vi "Find Ni-Scope digitizers.vi"(8 "Error In":errorcluster) -> (0 "Error Out":errorcluster, 2 "Device names out":string[](array[string]), 3 "Digitizers out":refnum<class "Pulse Driver.lvclass">[](array[class]))   [LabVIEW 2016, in "Ni-Scope Digitizer.lvclass"]
uses:
  Ni-Scope Digitizer.lvclass
  Instruments/Pulse Driver/Pulse Driver.lvclass
  C:/github/NHMFL_Core/Libraries/Instruments/Pulse Driver/Pulse Driver.lvclass
  Ni-Scope Digitizer.lvclass/Ni-Scope Digitizer.ctl
  Write Device name.vi
  <instrlib>/niModInst/niModInst Get Installed Device Attribute (String).vi
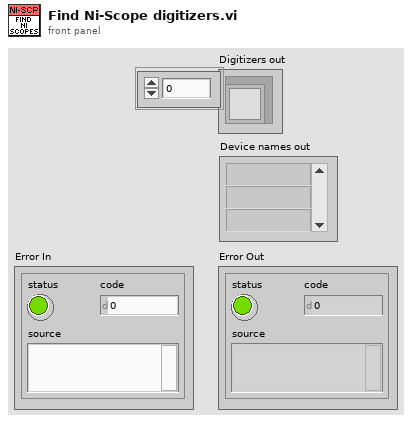
[diagram p1: front panel]
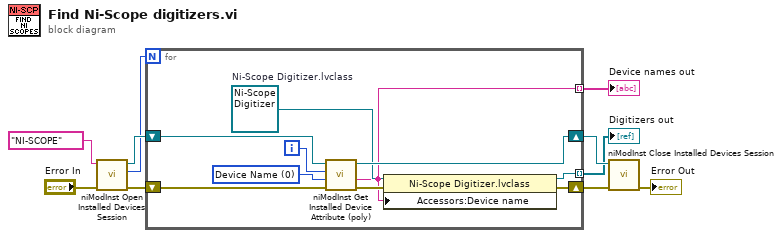
[diagram p0: block diagram]
diagram:
  n1 = call <instrlib>:"niModInst Open Installed Devices Session.vi"("error in (no error)"="Error In", "driver"="NI-SCOPE") -> ("error out"=w6:errorcluster, "device count"=w7:i32, "session"=w8:refnum<k20>)  [unwired: 7 in]
  n2 = for {
    N: w7 -> [_]
    shift-right: [w13] -> w4
    shift-left: w6 -> [w17]
    shift-right: [w18] -> w5
    shift-left: w8 -> [w19]
    tunnel: [w12] -> w2 mode=indexing
    tunnel: [w11] -> w1 mode=indexing
    i -> [w20]
    w15 = refnum<class "Ni-Scope Digitizer.lvclass"> refnum  # Ni-Scope Digitizer.lvclass
    w16 = 0 items=["Device Name", "Device Model", "Serial Number"] ("attribute ID")
    n3 = call-poly <instrlib>:"niModInst Get Installed Device Attribute (poly).vi"("error in (no error)"=w17, "attribute ID"=w16, "index in"=w20, "session in"=w19) -> ("error out"=w14:errorcluster, "attribute value"=w11:string, "session out"=w18:refnum<k20>)  [unwired: 5 out]
    n4 = property class="Ni-Scope Digitizer.lvclass"(reference=w15, error in=w14, "Accessors:Device name"=w11) -> (reference out=w12:refnum<class "Ni-Scope Digitizer.lvclass">, error out=w13:errorcluster)
  }
  "Digitizers out" <- w2
  "Device names out" <- w1
  n5 = call <instrlib>:"niModInst Close Installed Devices Session.vi"("error in (no error)"=w4, "session"=w5) -> ("error out"=→"Error Out":errorcluster)  [unwired: 9 out]
